vi "Add Items to Graph.vi"(7 "Depth Limit (12)":i32=12, 9 "Parent Index (None)":i32=-1, 10 "Items":variant[](array[variant]), 11 "Graph In":T1[](array[typedef])) -> (3 "Graph":T1[](array[typedef]))   [LabVIEW 2020, in "TypeGraph.lvlib"]
uses:
  TypeGraph.lvlib
  Type Reflection Item.ctl
  <vilib>/Utility/Data Type/Type Definitions/Data Type.ctl
  <vilib>/Utility/Data Type/NI_Data Type.lvlib
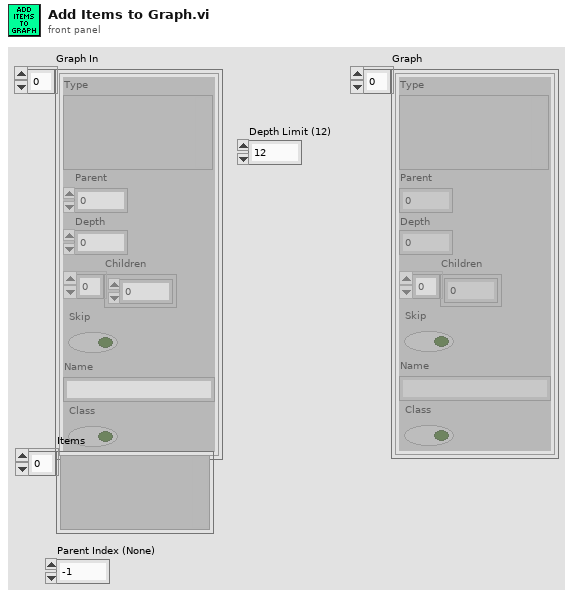
[diagram p1: front panel]
types:
  T1 = typedef "TypeGraph.lvlib/Type Reflection Item.ctl" = cluster{"Type":variant, "Parent":i32, "Depth":i32, "Children":i32[], "Skip":bool, "Name":string, "Class":bool}
  T2 = typedef "NI_Data Type.lvlib/Data Type.ctl" = enum8{"Invalid Type", "Void", "I8", "I16", "I32", "I64", "U8", "U16", "U32", "U64", "Single Float", "Double Float", "Extended Float", "Single Complex", "Double Complex", "Extended Complex", "Enum U8", "Enum U16", "Enum U32", "Enum U64", "Single Float With Unit", "Double Float With Unit", "Extended Float With Unit", "Single Complex with Unit", "Double Complex with Unit", "Extended Complex with Unit", "Boolean", "String", "Path", "Picture", "Tag", "Array", "Cluster", "Variant", "LV Variant", "Waveform", "Timestamp", "Digital Waveform", "Digital Data", "ExpressData", "Refnum", "External Data", "VI", "Poly VI", "LabVIEW Class Instance", "Fixed Point", "Set Collection", "Map Collection"}
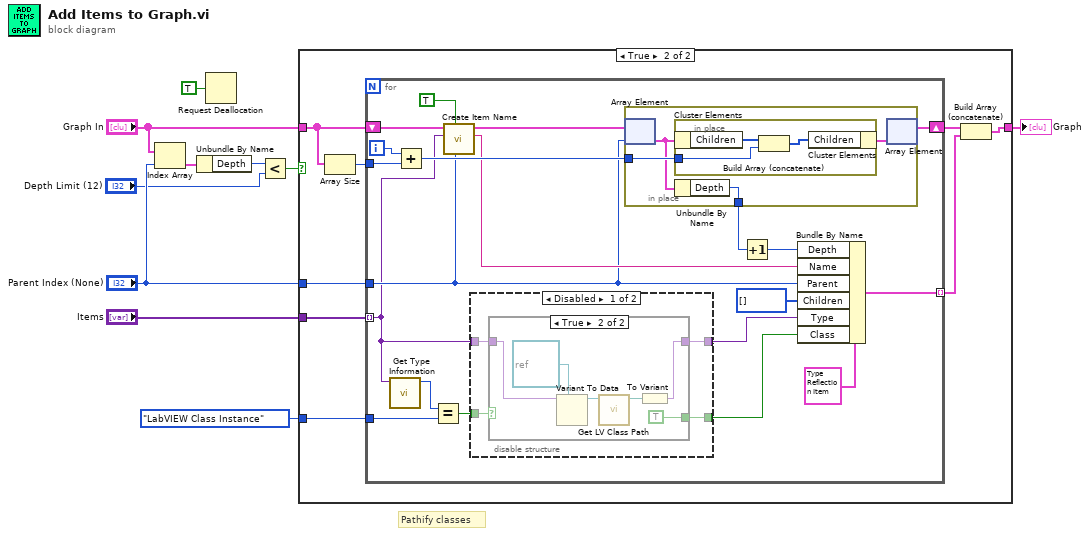
[diagram p0: block diagram]
diagram:
  # "Pathify classes"
  n1 = Index Array(array="Graph In", index="Parent Index (None)") -> (element=w6:T1)
  n2 = Unbundle By Name(w6) -> ("Depth"=w5:i32)
  n3 = Request Deallocation(TRUE ("flag")) -> ()
  n4 = Less?(x=w5, y="Depth Limit (12)") -> (x < y?=w3:bool)
  n5 = case shown="True" w3 {
    tunnel: [w11 w18] -> w10
    tunnel: "Items" -> [_ w17]
    tunnel: "Graph In" -> [w11 w14]
    tunnel: "Parent Index (None)" -> [_ w13]
    tunnel: Data_Type."LabVIEW Class Instance" ("y") -> [_ w12]
    frame False {
      # "Already at max depth, don't add more items."
    }
    frame True {
      n6 = Array Size(array=w14) -> (size(s)=w15:i32)
      n7 = for {
        tunnel: w13 -> [w27]
        tunnel: [w38] -> w19 mode=indexing
        tunnel: w17 -> [w22] mode=indexing
        shift-right: [w32] -> w16
        shift-left: w14 -> [w30]
        tunnel: w15 -> [w37]
        tunnel: w12 -> [w24]
        i -> [w36]
        n8 = call <vilib>:"Get Type Information.vi"("variant"=w22) -> ("type"=w25:T2)  [unwired: 6 in, 4 out]
        n9 = Add(x=w36, y=w37) -> (x+y=w35:i32)
        n10 = Equal?(x=w25, y=w24) -> (x = y?=w23:bool)
        n11 = call "Create Item Name.vi"("Parent"=w27, "Hide Full Name? (F)"=TRUE, "Type"=w22, "Item Graph In"=w30) -> ("Name"=w28:string, "Item Graph"=w29:T1[])  [unwired: 6 in]
        n12 = disable-structure shown="Disabled" {
          disable-tunnel: w23 -> [w43 w51]
          disable-tunnel: w22 -> [w42 w52]
          disable-tunnel: [w41 w52] -> w21
          disable-tunnel: [w40 w51] -> w20
          frame Disabled {
            n13 = case shown="True" w43 {
              tunnel: w42 -> [w44 w50]
              tunnel: [w44 w46] -> w41
              tunnel: [_ TRUE] -> w40
              frame False {
              }
              frame True {
                n14 = Variant To Data(type=refnum<class> refnum ("LabVIEW Object"), Variant=w50) -> (data=w48:refnum<class>)  [unwired: 1 in, 1 out]
                n15 = call <vilib>:"Get LV Class Path.vi"("object"=w48) -> ("class path"=w47:path)  [unwired: 9 in, 1 out]
                n16 = To Variant(anything=w47) -> (Variant=w46:variant)
              }
            }
          }
          frame Enabled {
          }
        }
        n17 = in-place {
          in-place-border: w35 -> [w56]
          in-place-border: [w53] -> w34
          n18 = in-place-array #1(w29, w27) -> (w54:T1)
          n19 = in-place {
            in-place-border: w56 -> [w58]
            n20 = in-place-cluster #2(w54) -> ("Children"=w59:i32[])
            n21 = Build Array (concatenate)(w59, w58) -> (w57:i32[])
            n22 = in-place-cluster #2("Children"=w57) -> (w55:T1)
          }
          n23 = Unbundle By Name(w54) -> ("Depth"=w53:i32)
          n24 = in-place-array #1(w55) -> (w32:T1[])  [unwired: 1 out]
        }
        n25 = Increment(x=w34) -> (x+1=w31:i32)
        n26 = Bundle By Name(cluster=T1 {"Type"=variant, "Parent"=-1, "Depth"=0, "Children"=[], "Skip"=FALSE, "Name"="", "Class"=FALSE} ("Type Reflection Item"), "Depth"=w31, "Name"=w28, "Parent"=w27, "Children"=i32[] [], "Type"=w21, "Class"=w20) -> (w38:T1)
      }
      n27 = Build Array (concatenate)(w16, w19) -> (w18:T1[])
    }
  }
  "Graph" <- w10
